vi "Filter Control Mouse Down Event.vi"(8 "error in (no error)":errorcluster, 10 "ControlMouseDownMsg":refnum<class "ControlMouseDownMsg.lvclass">, 11 "Test Executive Builder Event Filter in":refnum<class "Test Executive Builder Event Filter.lvclass">) -> (0 "error out":errorcluster, 1 "Discard?":bool, 2 "Filtered Event Data":T1, 3 "Test Executive Builder Event Filter out":refnum<class "Test Executive Builder Event Filter.lvclass">, 5 "Data Filtered?":bool)   [LabVIEW 2017, in "Test Executive Builder Event Filter.lvclass"]
uses:
  Test Executive Builder Event Filter.lvclass
  <vilib>/gpm_packages/@cs/mva-viewable/Source/ActorEvents/IEventAggregator Messages/ControlMouseDownMsg/ControlMouseDownMsg.lvclass
  Test Executive Builder View Messages/Handle Mouse Down Msg/Handle Mouse Down Msg.lvclass
  Application Dependencies/Mouse Down Filtered Event Data.ctl
  <vilib>/gpm_packages/@cs/actor-framework-messages/Source/RoundTripMessage/RoundTripMessage.lvclass
  C:/Users/jonmc/Documents/Git/Test Executive Builder/gpm_packages/@cs/actor-framework-messages/Source/RoundTripMessage/RoundTripMessage.lvclass
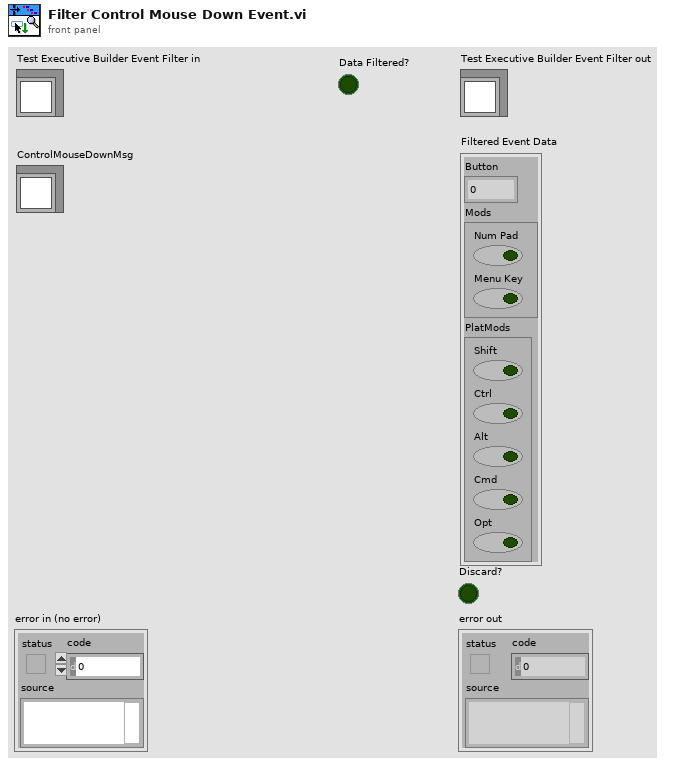
[diagram p1: front panel]
types:
  T1 = cluster{"Button":u16, "Mods":cluster{"Num Pad":bool, "Menu Key":bool}, "PlatMods":cluster{"Shift":bool, "Ctrl":bool, "Alt":bool, "Cmd":bool, "Opt":bool}}
  T2 = typedef "Mouse Down Filtered Event Data.ctl" = cluster{"Button":u16, "Mods":cluster{"Num Pad":bool, "Menu Key":bool}, "PlatMods":cluster{"Shift":bool, "Ctrl":bool, "Alt":bool, "Cmd":bool, "Opt":bool}, "Data Filtered?":bool, "Discard?":bool}
  T3 = typedef "LVPoint32TypeDef.ctl" = cluster{"Horizontal":i32, "Vertical":i32}
  T4 = cluster{"Shift":bool, "Ctrl":bool, "Alt":bool, "Cmd":bool, "Opt":bool}
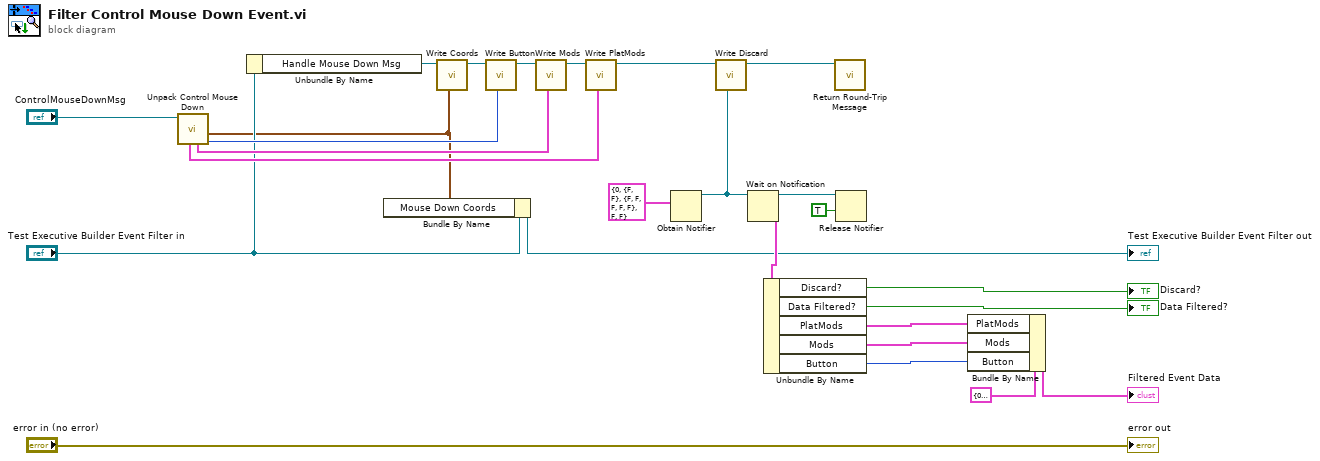
[diagram p0: block diagram]
diagram:
  n1 = call <vilib>:"Unpack Control Mouse Down.vi"("ControlMouseDownMsg"="ControlMouseDownMsg") -> ("Button"=w17:u16, "Coords"=w2:T3, "Mods"=w14:cluster{"Double Click":bool, "Menu Key":bool}, "PlatMods"=w13:T4)  [unwired: 4 in, 3 out]
  n2 = Unbundle By Name("Test Executive Builder Event Filter in") -> ("Handle Mouse Down Msg"=w22:refnum<class "Handle Mouse Down Msg.lvclass">)
  n3 = Bundle By Name(cluster="Test Executive Builder Event Filter in", "Mouse Down Coords"=w2) -> (→"Test Executive Builder Event Filter out":refnum<class "Test Executive Builder Event Filter.lvclass">)
  n4 = call "Write Coords.vi"("Coordinates"=w2, "Handle Mouse Down Msg in"=w22) -> ("Handle Mouse Down Msg out"=w21:refnum<class "Handle Mouse Down Msg.lvclass">)  [unwired: 9 in]
  n5 = call "Write Button.vi"("Button"=w17, "Handle Mouse Down Msg in"=w21) -> ("Handle Mouse Down Msg out"=w20:refnum<class "Handle Mouse Down Msg.lvclass">)  [unwired: 9 in]
  n6 = call "Write Mods.vi"("Mods"=w14, "Handle Mouse Down Msg in"=w20) -> ("Handle Mouse Down Msg out"=w19:refnum<class "Handle Mouse Down Msg.lvclass">)  [unwired: 9 in]
  n7 = call "Write PlatMods.vi"("PlatMods"=w13, "Handle Mouse Down Msg in"=w19) -> ("Handle Mouse Down Msg out"=w18:refnum<class "Handle Mouse Down Msg.lvclass">)  [unwired: 9 in]
  n8 = Obtain Notifier(notification data type=T2 {"Button"=0, "Mods"={"Num Pad"=FALSE, "Menu Key"=FALSE}, "PlatMods"={"Shift"=FALSE, "Ctrl"=FALSE, "Alt"=FALSE, "Cmd"=FALSE, "Opt"=FALSE}, "Data Filtered?"=FALSE, "Discard?"=FALSE} ("Mouse Down Filtered Event Data")) -> (notifier out=w11:refnum<notifier>)  [unwired: 3 in, 2 out]
  n9 = call "Write Discard.vi"("Mouse Down Filtered Event Data"=w11, "Handle Mouse Down Msg in"=w18) -> ("Handle Mouse Down Msg out"=w1:refnum<class "Handle Mouse Down Msg.lvclass">)  [unwired: 9 in]
  n10 = Wait on Notification(notifier=w11) -> (notifier out=w24:refnum<notifier>, notification=w10:T2)  [unwired: 3 in, 2 out]
  n11 = Unbundle By Name(w10) -> ("Discard?"=→"Discard?":bool, "Data Filtered?"=→"Data Filtered?":bool, "PlatMods"=w7:T4, "Mods"=w6:cluster{"Num Pad":bool, "Menu Key":bool}, "Button"=w5:u16)
  n12 = call <vilib>:"Return Round-Trip Message.vi"("RoundTripMessage In"=w1) -> ()  [unwired: 10 in, 1 out]
  n13 = Release Notifier(notifier=w24, force destroy? (F)=TRUE) -> ()  [unwired: 1 in, 3 out]
  n14 = Bundle By Name(cluster=T1 {"Button"=0, "Mods"={"Num Pad"=FALSE, "Menu Key"=FALSE}, "PlatMods"={"Shift"=FALSE, "Ctrl"=FALSE, "Alt"=FALSE, "Cmd"=FALSE, "Opt"=FALSE}} ("Filtered Event Data"), "PlatMods"=w7, "Mods"=w6, "Button"=w5) -> (→"Filtered Event Data":T1)
  "error out" <- "error in (no error)"
